vi "Teleop.vi"(10 "Match Info":T1={"Autonomous Elapsed Seconds"=0.0, "TeleOp Elapsed Seconds"=0.0, "Disabled Elapsed Seconds"=0.0, "Visited Autonomous"=FALSE, "Visited TeleOp"=FALSE, "Visited Disabled"=FALSE, "Autonomous Settings"={"Autonomous Style"=enum."Independent", "VI Refnum"=refnum}}, 11 "Call Context":T2) -> ()   [LabVIEW 2020]
doc: "This VI is called for each TeleOp packet received from the DS where the robot is not disabled. It is often used to read from the joysticks and update I/O or to update setpoints for timed control loops. It should complete and return within 20 milliseconds or it may miss DS packets."
uses:
  <vilib>/Rock Robotics/WPI/DriverStation/WPI_DriverStationDerivedRobotMode.ctl
  <vilib>/Rock Robotics/WPI/DriverStation/WPI_DriverStationMatch Info.ctl
  <vilib>/Rock Robotics/WPI/Solenoid/WPI_SolenoidValue.ctl
  <vilib>/Rock Robotics/WPI/SafetyOutput/WPI_SafetyOutputConfigMenu.ctl
  <vilib>/Rock Robotics/WPI/ThirdParty/REV Robotics/REVLib/Typedef/Spark MAX Control Type.ctl
  <vilib>/Rock Robotics/WPI/Utilities/WPI_GetSetVariantRefNum.vi
  Global Sensor Reads.vi
  <vilib>/Rock Robotics/WPI/Solenoid/WPI_SolenoidSetEnum.vi
  Global Shooter Speed.vi
  <vilib>/Rock Robotics/Network Tables/NT Write Number.vi
  <vilib>/Rock Robotics/Network Tables/NT Read Number.vi
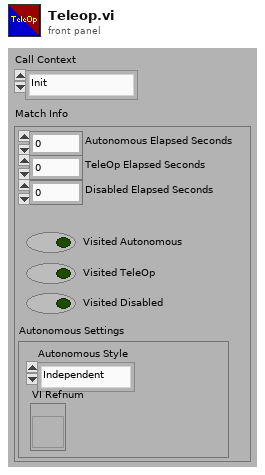
[diagram p1: front panel]
types:
  T1 = typedef "WPI_DriverStationMatch Info.ctl" = cluster{"Autonomous Elapsed Seconds":dbl, "TeleOp Elapsed Seconds":dbl, "Disabled Elapsed Seconds":dbl, "Visited Autonomous":bool, "Visited TeleOp":bool, "Visited Disabled":bool, "Autonomous Settings":cluster{"Autonomous Style":enum16{"Iterative", "Independent"}, "VI Refnum":refnum<vi>}}
  T2 = typedef "WPI_DriverStationDerivedRobotMode.ctl" = enum16{"Init", "Execute", "Stop"}
  T3 = typedef "WPI_SafetyOutputConfigMenu.ctl" = enum16{"Enable", "Disable"}
  T4 = typedef "WPI_SolenoidValue.ctl" = enum16{"Off", "On", "Forward", "Reverse"}
  T5 = typedef "Joystick_Controls.ctl" = cluster{"Pilot Left Joystick X":dbl, "Pilot Left Joystick Y":dbl, "Pilot X Button":bool, "Pilot Circle Button":bool, "Pilot Square Button":bool, "Pilot Triangle Button":bool, "Pilot Left Bumper":bool, "Pilot Right Bumper":bool, "Pilot Share Button":bool, "Pilot Options Button":bool, "Pilot Left Joystick Press":bool, "Pilot Right Joystick Press":bool, "Pilot Left Trigger":dbl, "Pilot Right Joystick X":dbl, "Pilot Right Joystick Y":dbl, "Pilot Right Trigger":dbl, "Copilot Left Joystick X":dbl, "Copilot Left Joystick Y":dbl, "Copilot A Button":bool, "Copilot B Button":bool, "Copilot X Button":bool, "Copilot Y Button":bool, "Copilot Left Bumper":bool, "Copilot Right Bumper":bool, "Copilot View Button":bool, "Copilot Menu Button":bool, "Copilot Left Joystick Press":bool, "Copilot Right Joystick Press":bool, "Copilot Left Trigger":dbl, "Copilot Right Joystick X":dbl, "Copilot Right Joystick Y":dbl, "Copilot Right Trigger":dbl, "Pilot D-pad North":bool, "Pilot D-pad South":bool, "Pilot D-pad East":bool, "Pilot D-pad West":bool, "Pilot D-pad NE ":bool, "Pilot D-pad SE":bool, "Pilot D-pad SW":bool, "Pilot D-pad NW":bool, "CoPilot D-pad North":bool, "CoPilot D-pad South":bool, "CoPilot D-pad East":bool, "CoPilot D-pad West":bool, "CoPilot D-pad NE":bool, "CoPilot D-pad SE":bool, "CoPilot D-pad SW":bool, "CoPilot D-pad NW":bool, "Pilot Left Trigger Pressed":bool, "Pilot Right Trigger Pressed":bool, "CoPilot Left Trigger Pressed":bool, "CoPilot Right Trigger Pressed":bool, "Pilot Left Trigger Firmly":bool, "Pilot Right Trigger Firmly":bool, "Pilot Touchpad":bool, "Pilot PS Button":bool}
  T6 = typedef "WPI_JoystickDevRef.ctl" = cluster{"Device":T7}
  T7 = typedef "WPI_JoystickDeviceEnum.ctl" = enum16{"USB 0", "USB 1", "USB 2", "USB 3", "USB 4", "USB 5"}
  T8 = typedef "WPI_MotorControlDeviceRef.ctl" = cluster{"DeviceStatus":errorcluster, "Type":T9, "PWM":cluster{"PWM Channel":T10, "DeadBand":T11}, "CAN":cluster{"Device Number":u8, "SetOutput VI Ref":variant, "GetOutput VI Ref":variant, "Enable VI Ref":variant, "Disable VI Ref":variant, "Data":variant}, "Invert":bool, "DIO PWM":cluster{"PWM \"Enable\" Channel":T10, "DIOChannel":T12, "PWM Rate":dbl}}
  T9 = typedef "WPI_MotorControlType.ctl" = enum16{"PWM", "CAN", "DIO PWM"}
  T10 = typedef "FPGA_DIOPWMChannel.ctl" = enum8{"PWM 0", "PWM 1", "PWM 2", "PWM 3", "PWM 4", "PWM 5", "PWM 6", "PWM 7", "PWM 8", "PWM 9", "PWM MXP 0", "PWM MXP 1", "PWM MXP 2", "PWM MXP 3", "PWM MXP 4", "PWM MXP 5", "PWM MXP 6", "PWM MXP 7", "PWM MXP 8", "PWM MXP 9", "Invalid"}
  T11 = typedef "WPI_PWMDeadband.ctl" = cluster{"Name":string, "maxPositivePwm":i32, "minPositivePwm":i32, "centerPwm":i32, "maxNegativePwm":i32, "minNegativePwm":i32, "angularRange":u16}
  T12 = typedef "FPGA_DIOChannel.ctl" = enum8{"DIO 0", "DIO 1", "DIO 2", "DIO 3", "DIO 4", "DIO 5", "DIO 6", "DIO 7", "DIO 8", "DIO 9", "DIO MXP 0", "DIO MXP 1", "DIO MXP 2", "DIO MXP 3", "DIO MXP 4", "DIO MXP 5", "DIO MXP 6", "DIO MXP 7", "DIO MXP 8", "DIO MXP 9", "DIO MXP 10", "DIO MXP 11", "DIO MXP 12", "DIO MXP 13", "DIO MXP 14", "DIO MXP 15", "SPI Port CS1", "SPI Port CS2", "SPI Port CS3", "SPI Port MISO", "SPI Port MOSI", "Invalid"}
  T13 = typedef "Spark MAX Control Type.ctl" = enum16{"Percent VBus", "Voltage", "Velocity", "Position", "Smart Motion", "Current", "Smart Velocity"}
  T14 = typedef "WPI_RobotDriveDevRef.ctl" = cluster{"DevStatus":errorcluster, "Motors[]":T8[], "Square Inputs":bool, "Max Output":dbl}
  T15 = typedef "WPI_SolenoidDevRef.ctl" = cluster{"DevStatus":errorcluster, "Pneumatics Control Module":u8, "Forward Solenoid Channel":T16, "Reverse Solenoid Channel":T16}
  T16 = typedef "WPI_SolenoidChannel.ctl" = enum8{"Solenoid 0", "Solenoid 1", "Solenoid 2", "Solenoid 3", "Solenoid 4", "Solenoid 5", "Solenoid 6", "Solenoid 7", "Solenoid 8", "Solenoid 9", "Solenoid 10", "Solenoid 11", "Solenoid 12", "Solenoid 13", "Solenoid 14", "Solenoid 15", "Invalid"}
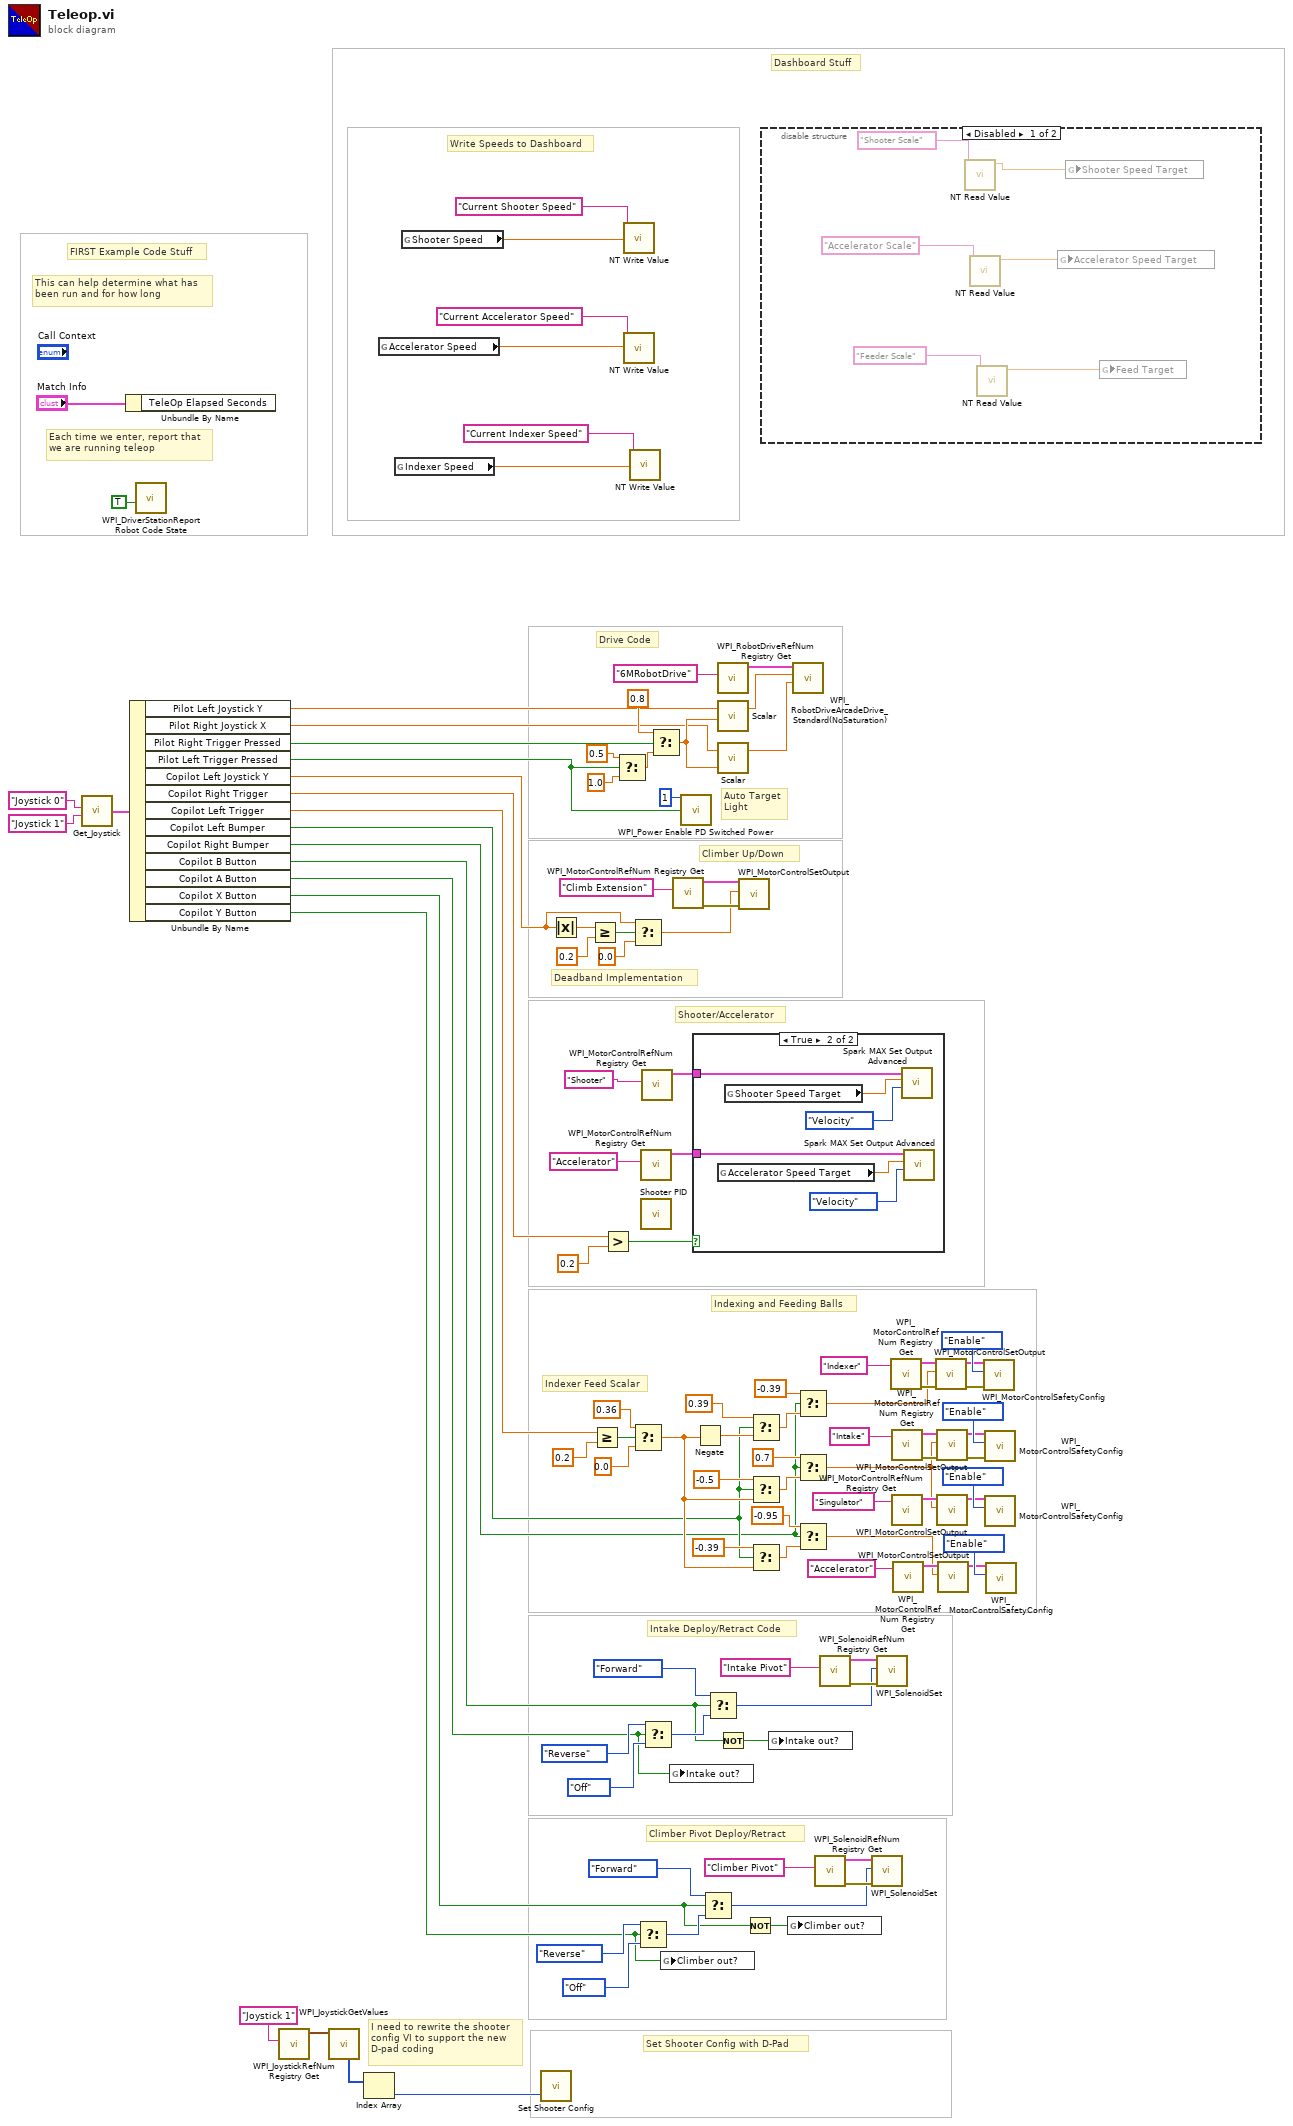
[diagram p0: block diagram]
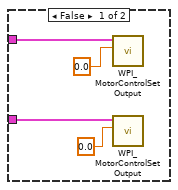
[diagram p2: hidden frame]
diagram:
  # "I need to rewrite the shooter\nconfig VI to support the new\nD-pad coding"
  # "Dashboard Stuff"
  # "FIRST Example Code Stuff"
  # "Indexing and Feeding Balls"
  # "Indexer Feed Scalar"
  # "Set Shooter Config with D-Pad"
  # "Shooter/Accelerator"
  # "Climber Up/Down"
  # "Deadband Implementation"
  # "Climber Pivot Deploy/Retract"
  # "Intake Deploy/Retract Code"
  # "Auto Target\nLight"
  # "Drive Code"
  # "Write Speeds to Dashboard"
  # "Each time we enter, report that\nwe are running teleop"
  # "This can help determine what has\nbeen run and for how long"
  n1 = call "Get_Joystick.vi"("Joystick_One"="Joystick 0" ("refnum name"), "Joystick_Two"="Joystick 1" ("refnum name")) -> ("Joystick_Out"=w19:T5)  [unwired: 5 in]
  n2 = Unbundle By Name("Match Info") -> ()  [unwired: 1 out]
  n3 = Unbundle By Name(w19) -> ("Pilot Left Joystick Y"=w18:dbl, "Pilot Right Joystick X"=w17:dbl, "Pilot Right Trigger Pressed"=w15:bool, "Pilot Left Trigger Pressed"=w16:bool, "Copilot Left Joystick Y"=w14:dbl, "Copilot Right Trigger"=w13:dbl, "Copilot Left Trigger"=w12:dbl, "Copilot Left Bumper"=w11:bool, "Copilot Right Bumper"=w10:bool, "Copilot B Button"=w7:bool, "Copilot A Button"=w9:bool, "Copilot X Button"=w4:bool, "Copilot Y Button"=w6:bool)
  n4 = call <vilib>:"WPI_DriverStationReport Robot Code State.vi"("TeleOp"=TRUE ("Autonomous")) -> ()  [unwired: 10 in, 1 out]
  n5 = call <vilib>:"WPI_JoystickRefNum Registry Get.vi"("refnum name"="Joystick 1") -> ("JoystickDevRef"=w102:T6)  [unwired: 1 in, 9 out]
  n6 = call <vilib>:"WPI_JoystickGetValues.vi"("JoystickDevRef"=w102) -> ("POVs"=w61:i16[])  [unwired: 6 in, 4 out]
  n7 = Index Array(array=w61) -> (element=w60:i16)  [unwired: 1 in]
  n8 = global read "Global Sensor Reads.vi" "Accelerator Speed"() -> (w2:dbl)
  n9 = global read "Global Sensor Reads.vi" "Indexer Speed"() -> (w1:dbl)
  n10 = global read "Global Sensor Reads.vi" "Shooter Speed"() -> (w3:dbl)
  n11 = call "Set Shooter Config.vi"("POV Joystick Input"=w60) -> ()  [unwired: 3 in]
  n12 = Absolute Value(x=w14) -> (abs(x)=w75:dbl)
  n13 = Greater Or Equal?(x=w75, y=0.2) -> (x >= y?=w73:bool)
  n14 = Greater Or Equal?(x=w12, y=0.2) -> (x >= y?=w58:bool)
  n15 = Greater?(x=w13, y=0.2) -> (0:w64:bool)
  n16 = Select(t=0.5, s=w16, f=1.0) -> (s? t:f=w95:dbl)
  n17 = call-poly <vilib>:"NT Write Value.vi"("Numeric"=w3, "Name"="Current Shooter Speed") -> ()  [unwired: 9 in, 1 out]
  n18 = call-poly <vilib>:"NT Write Value.vi"("Numeric"=w2, "Name"="Current Accelerator Speed") -> ()  [unwired: 9 in, 1 out]
  n19 = call-poly <vilib>:"NT Write Value.vi"("Numeric"=w1, "Name"="Current Indexer Speed") -> ()  [unwired: 9 in, 1 out]
  n20 = Select(t=w14, s=w73, f=0.0) -> (s? t:f=w68:dbl)
  n21 = Select(t=0.36, s=w58, f=0.0) -> (s? t:f=w48:dbl)
  n22 = Select(t=WPI_SolenoidValue."Reverse" ("Value"), s=w6, f=WPI_SolenoidValue."Off" ("Value")) -> (s? t:f=w78:T4)
  n23 = call <vilib>:"WPI_MotorControlRefNum Registry Get.vi"("refnum name"="Accelerator") -> ("MotorControlDevRef"=w62:T8)  [unwired: 9 in, 1 out]
  n24 = call "Shooter PID.vi"() -> ()  [unwired: 12 in]
  n25 = call <vilib>:"WPI_MotorControlRefNum Registry Get.vi"("refnum name"="Shooter") -> ("MotorControlDevRef"=w63:T8)  [unwired: 9 in, 1 out]
  n26 = Select(t=WPI_SolenoidValue."Reverse" ("Value"), s=w9, f=WPI_SolenoidValue."Off" ("Value")) -> (s? t:f=w86:T4)
  n27 = Select(t=0.8, s=w15, f=w95) -> (s? t:f=w96:dbl)
  n28 = global write "Global Sensor Reads.vi" "Climber out?"(w6) -> ()
  n29 = global write "Global Sensor Reads.vi" "Intake out?"(w9) -> ()
  n30 = call <vilib>:"WPI_MotorControlRefNum Registry Get.vi"("refnum name"="Climb Extension") -> ("error out"=w70:errorcluster, "MotorControlDevRef"=w71:T8)  [unwired: 9 in]
  n31 = call <vilib>:"WPI_Power Enable PD Switched Power.vi"("Power Distribution (def)"=u8 1, "Switch Channel Value"=w16) -> ()  [unwired: 12 in, 2 out]
  n32 = case shown="True" w64 {
    tunnel: w63 -> [w112 w118]
    tunnel: w62 -> [w111 w115]
    frame False {
      n33 = call <vilib>:"WPI_MotorControlSetOutput.vi"("Output"=0.0, "MotorControlDevRef"=w112) -> ()  [unwired: 7 in, 3 out]
      n34 = call <vilib>:"WPI_MotorControlSetOutput.vi"("Output"=0.0, "MotorControlDevRef"=w111) -> ()  [unwired: 7 in, 3 out]
    }
    frame True {
      n35 = global read "Global Shooter Speed.vi" "Accelerator Speed Target"() -> (w114:dbl)
      n36 = global read "Global Shooter Speed.vi" "Shooter Speed Target"() -> (w117:dbl)
      n37 = call <vilib>:"Spark MAX Set Output Advanced.vi"("Control Mode"=Spark_MAX_Control_Type."Velocity", "Setpoint"=w117, "MotorControlDevRef"=w118) -> ()  [unwired: 7 in, 2 out]
      n38 = call <vilib>:"Spark MAX Set Output Advanced.vi"("Control Mode"=Spark_MAX_Control_Type."Velocity", "Setpoint"=w114, "MotorControlDevRef"=w115) -> ()  [unwired: 7 in, 2 out]
    }
  }
  n39 = Negate(x=w48) -> (-x=w55:dbl)
  n40 = Select(t=WPI_SolenoidValue."Forward" ("Value"), s=w4, f=w78) -> (s? t:f=w76:T4)
  n41 = Select(t=WPI_SolenoidValue."Forward" ("Value"), s=w7, f=w86) -> (s? t:f=w84:T4)
  n42 = call <vilib>:"WPI_RobotDriveRefNum Registry Get.vi"("refnum name"="6MRobotDrive") -> ("RobotDriveDevRef"=w100:T14)  [unwired: 1 in, 9 out]
  n43 = call "Scalar.vi"("Scalar"=w96, "Joystick Value"=w18) -> ("Final Joystick Value"=w99:dbl)  [unwired: 1 in]
  n44 = call "Scalar.vi"("Scalar"=w96, "Joystick Value"=w17) -> ("Final Joystick Value"=w98:dbl)  [unwired: 1 in]
  n45 = Not(x=w7) -> (.not. x?=w8:bool)
  n46 = call <vilib>:"WPI_MotorControlSetOutput.vi"("error in (no error)"=w70, "Output"=w68, "MotorControlDevRef"=w71) -> ()  [unwired: 6 in, 3 out]
  n47 = Not(x=w4) -> (.not. x?=w5:bool)
  n48 = Select(t=0.39, s=w11, f=w55) -> (s? t:f=w54:dbl)
  n49 = Select(t=-0.5, s=w11, f=w48) -> (s? t:f=w50:dbl)
  n50 = Select(t=-0.39, s=w11, f=w48) -> (s? t:f=w46:dbl)
  n51 = disable-structure shown="Disabled" {
    frame Disabled {
      n52 = call-poly <vilib>:"NT Read Value.vi"("Name"="Shooter Scale") -> ("Numeric"=w123:dbl)  [unwired: 9 in, 1 out]
      n53 = call-poly <vilib>:"NT Read Value.vi"("Name"="Accelerator Scale") -> ("Numeric"=w121:dbl)  [unwired: 9 in, 1 out]
      n54 = call-poly <vilib>:"NT Read Value.vi"("Name"="Feeder Scale") -> ("Numeric"=w119:dbl)  [unwired: 9 in, 1 out]
      n55 = global write "Global Shooter Speed.vi" "Accelerator Speed Target"(w121) -> ()
      n56 = global write "Global Shooter Speed.vi" "Shooter Speed Target"(w123) -> ()
      n57 = global write "Global Shooter Speed.vi" "Feed Target"(w119) -> ()
    }
    frame Enabled {
    }
  }
  n58 = global write "Global Sensor Reads.vi" "Intake out?"(w8) -> ()
  n59 = global write "Global Sensor Reads.vi" "Climber out?"(w5) -> ()
  n60 = call <vilib>:"WPI_RobotDriveArcadeDrive_Standard(NoSaturation).vi"("Y axis value"=w98, "X axis value"=w99, "RobotDriveDevRef"=w100) -> ()  [unwired: 1 in, 8 out]
  n61 = Select(t=-0.39, s=w10, f=w54) -> (s? t:f=w38:dbl)
  n62 = Select(t=0.7, s=w10, f=w50) -> (s? t:f=w27:dbl)
  n63 = Select(t=-0.95, s=w10, f=w46) -> (s? t:f=w22:dbl)
  n64 = call <vilib>:"WPI_SolenoidRefNum Registry Get.vi"("refnum name"="Climber Pivot") -> ("error out"=w81:errorcluster, "SolenoidDevRef"=w83:T15)  [unwired: 9 in]
  n65 = call <vilib>:"WPI_SolenoidRefNum Registry Get.vi"("refnum name"="Intake Pivot") -> ("error out"=w89:errorcluster, "SolenoidDevRef"=w91:T15)  [unwired: 9 in]
  n66 = call-poly <vilib>:"WPI_SolenoidSet.vi"("error in (no error)"=w81, "Value"=w76, "SolenoidDevRef"=w83) -> ()  [unwired: 7 in, 2 out]
  n67 = call-poly <vilib>:"WPI_SolenoidSet.vi"("error in (no error)"=w89, "Value"=w84, "SolenoidDevRef"=w91) -> ()  [unwired: 7 in, 2 out]
  n68 = call <vilib>:"WPI_MotorControlRefNum Registry Get.vi"("refnum name"="Indexer") -> ("error out"=w40:errorcluster, "MotorControlDevRef"=w44:T8)  [unwired: 9 in]
  n69 = call <vilib>:"WPI_MotorControlRefNum Registry Get.vi"("refnum name"="Intake") -> ("error out"=w33:errorcluster, "MotorControlDevRef"=w37:T8)  [unwired: 9 in]
  n70 = call <vilib>:"WPI_MotorControlRefNum Registry Get.vi"("refnum name"="Singulator") -> ("MotorControlDevRef"=w31:T8)  [unwired: 9 in, 1 out]
  n71 = call <vilib>:"WPI_MotorControlRefNum Registry Get.vi"("refnum name"="Accelerator") -> ("MotorControlDevRef"=w26:T8)  [unwired: 9 in, 1 out]
  n72 = call <vilib>:"WPI_MotorControlSetOutput.vi"("error in (no error)"=w40, "Output"=w38, "MotorControlDevRef"=w44) -> ("error out"=w39:errorcluster, "MotorControlDevRef"=w41:T8)  [unwired: 6 in, 1 out]
  n73 = call <vilib>:"WPI_MotorControlSetOutput.vi"("error in (no error)"=w33, "Output"=w27, "MotorControlDevRef"=w37) -> ("error out"=w32:errorcluster, "MotorControlDevRef"=w34:T8)  [unwired: 6 in, 1 out]
  n74 = call <vilib>:"WPI_MotorControlSetOutput.vi"("Output"=w27, "MotorControlDevRef"=w31) -> ("MotorControlDevRef"=w28:T8)  [unwired: 7 in, 2 out]
  n75 = call <vilib>:"WPI_MotorControlSetOutput.vi"("Output"=w22, "MotorControlDevRef"=w26) -> ("MotorControlDevRef"=w23:T8)  [unwired: 7 in, 2 out]
  n76 = call <vilib>:"WPI_MotorControlSafetyConfig.vi"("error in (no error)"=w39, "mode"=WPI_SafetyOutputConfigMenu."Enable", "MotorControlDevRef"=w41) -> ()  [unwired: 7 in, 2 out]
  n77 = call <vilib>:"WPI_MotorControlSafetyConfig.vi"("error in (no error)"=w32, "mode"=WPI_SafetyOutputConfigMenu."Enable", "MotorControlDevRef"=w34) -> ()  [unwired: 7 in, 2 out]
  n78 = call <vilib>:"WPI_MotorControlSafetyConfig.vi"("mode"=WPI_SafetyOutputConfigMenu."Enable", "MotorControlDevRef"=w28) -> ()  [unwired: 8 in, 2 out]
  n79 = call <vilib>:"WPI_MotorControlSafetyConfig.vi"("mode"=WPI_SafetyOutputConfigMenu."Enable", "MotorControlDevRef"=w23) -> ()  [unwired: 8 in, 2 out]
